vi "action.vi"(0 "HGF_ThreadTaskOnce":refnum<class "HGF_TaskOnce.lvclass">, 5 "error in (no error)":errorcluster, 8 "HGF_ThreadWorker":refnum<class "HGF_ThreadWorker.lvclass">) -> (10 "dup HGF_ThreadWorker":refnum<class "HGF_ThreadWorker.lvclass">, 14 "dup HGF_ThreadTaskOnce":refnum<class "HGF_TaskOnce.lvclass">, 19 "error out":errorcluster)   [LabVIEW 2014, in "HGF_BaseClasses.lvlib" / "HGF_TaskOnce.lvclass"]
doc: "This is a dynamic dispatch VI that is called from Visitor.visit(). It will call member VIs of Visitable to perform the requested action which means: calling public methods of Visitable child class.\n\n<B>Hint:</B> This method is abstract and need to be implemented by child classes."
uses:
  HGF_TaskOnce.lvclass
  HGF_ThreadTask/HGF_ThreadTask.lvclass
  HGF_Visitor/HGF_Visitor.lvclass
  HGF_Event/HGF_Event.lvclass
  HGF_ThreadWorker/HGF_ThreadWorker.lvclass
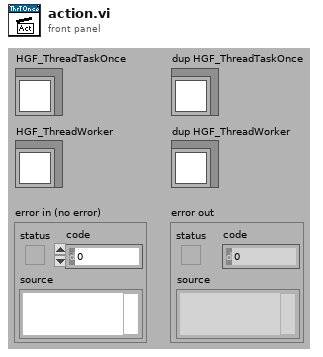
[diagram p1: front panel]
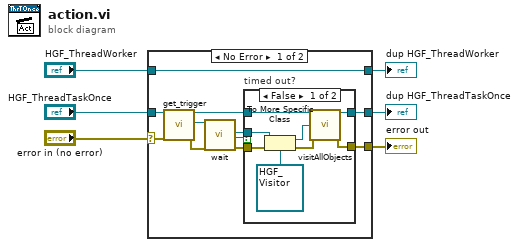
[diagram p0: block diagram]
diagram:
  n1 = case shown="No Error" "error in (no error)" {
    selector: "error in (no error)" -> [w16 w29]
    tunnel: "HGF_ThreadTaskOnce" -> [w17 w30]
    tunnel: [w13 w30] -> w5
    tunnel: [w11 w29] -> w4
    tunnel: [w10 w28] -> w2
    tunnel: "HGF_ThreadWorker" -> [w10 w28]
    frame No Error {
      n2 = call "get_trigger.vi"("HGF_ThreadTask"=w17, "error in (no error)"=w16) -> ("dup HGF_ThreadTask"=w12:refnum<class "HGF_TaskOnce.lvclass">, "trigger"=w15:refnum<class "HGF_Event.lvclass">, "error out"=w14:errorcluster)  [unwired: 15 out]
      n3 = call-dynamic "wait.vi"("HGF_Event"=w15, "error in (no error)"=w14) -> ("Object"=w7:refnum<class>, "timed out"=w9:bool, "error out"=w8:errorcluster)  [unwired: 2 in, 13 out]
      n4 = case "timed out?" shown="False" w9 {
        tunnel: [w21 w27] -> w13
        tunnel: w12 -> [w22 w27]
        tunnel: w8 -> [w25 w26]
        tunnel: [w18 w26] -> w11
        tunnel: w7 -> [w24 _]
        frame False {
          n5 = To More Specific Class(target class=refnum<class "HGF_Visitor.lvclass"> refnum ("HGF_BaseClasses.lvlib:HGF_Visitor.lvclass"), reference=w24, error in=w25) -> (specific class reference=w19:refnum<class "HGF_Visitor.lvclass">, error out=w20:errorcluster)
          n6 = call-dynamic "visitAllObjects.vi"("HGF_ThreadTask"=w22, "HGF_Visitor"=w19, "error in (no error)"=w20) -> ("dup HGF_ThreadTask"=w21:refnum<class "HGF_TaskOnce.lvclass">, "error out"=w18:errorcluster)  [unwired: 11 out]
        }
        frame True {
        }
      }
    }
    frame Error {
    }
  }
  "error out" <- w4
  "dup HGF_ThreadTaskOnce" <- w5
  "dup HGF_ThreadWorker" <- w2
